vi "OpenCom.vi"(11 "error in (no error)":errorcluster) -> (15 "error out":errorcluster)   [LabVIEW 2009]
uses:
  <vilib>/Instr/_visa.llb/VISA Set IO Buffer Mask.ctl
  globals/VISAResourceName.vi
  <vilib>/Instr/_visa.llb/VISA Configure Serial Port (Instr).vi
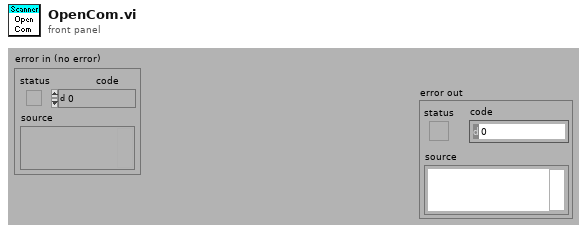
[diagram p1: front panel]
types:
  T1 = typedef "VISA Set IO Buffer Mask.ctl" = u16
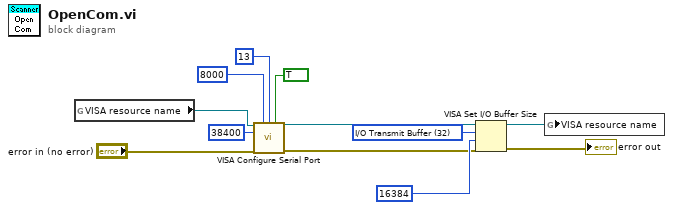
[diagram p0: block diagram]
diagram:
  w6 = T1 32 items=["I/O Receive Buffer"=16, "I/O Transmit Buffer"=32, "I/O Receive and Transmit Buffer"=48] ("Mask")
  n1 = global read "VISAResourceName.vi" "VISA resource name"() -> (w2:refnum<visa-resource-name>)
  n2 = call-poly "VISA Configure Serial Port"("VISA resource name"=w2, "timeout (10sec)"=u32 8000, "termination char\n(0xA = '\\n' = LF)"=u8 13 ("termination char\n(0xA = '\\n' = LF)"), "Enable Termination\nChar (T)"=TRUE ("Enable Termination\nChar (T)"), "baud rate (9600)"=u32 38400, "error in (no error)"="error in (no error)") -> ("VISA resource name out"=w7:refnum<visa-resource-name>, "error out"=w4:errorcluster)  [unwired: 8 in]
  n3 = VISA Set I/O Buffer Size(VISA resource name=w7, mask (16)=w6, size (4096)=u32 16384, error in (no error)=w4) -> (VISA resource name out=w8:refnum<visa-resource-name>, error out=→"error out":errorcluster)
  n4 = global write "VISAResourceName.vi" "VISA resource name"(w8) -> ()
